vi "Periodic Tasks.vi"(8 "error in":errorcluster) -> ()   [LabVIEW 2018]
doc: "This VI runs in parallel to other tasks. It can contain as many user-defined periodic loops as you need. These can carry out PID or other sorts of timed response."
uses:
  <vilib>/Rock Robotics/WPI/Utilities/WPI_GetSetVariantRefNum.vi
  Functions/Global Variables/reset gyro.vi
  <vilib>/Rock Robotics/WPI/ThirdParty/Sensors/ADIS16448 IMU/ADIS16448_IMU.lvlib
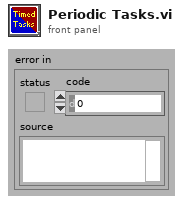
[diagram p1: front panel]
types:
  T1 = typedef "ADIS16448_IMU.lvlib/ADI_IMU_ADIS16448_IMUDevRef.ctl" = cluster{"DevStatus":errorcluster, "Handle":i32, "SPI Bus":T2, "Device Found":bool, "Device Ready":bool, "Yaw Axis":enum16{"X", "Y", "Z"}, "AHRS Algorithm":enum16{"Complementary", "Madgwick"}, "Serial":u16, "Lot ID 2":u16, "Lot ID 1":u16, "Bytes Per Sample":u16, "Calibrate On Open?":bool}
  T2 = typedef "spi_bus.ctl" = enum16{"SPI On-Board, CS0", "SPI On-Board, CS1", "SPI On-Board, CS2", "SPI On-Board, CS3", "SPI MXP", "Invalid"}
  T3 = typedef "WPI_JoystickDevRef.ctl" = cluster{"Device":T4}
  T4 = typedef "WPI_JoystickDeviceEnum.ctl" = enum16{"USB 0", "USB 1", "USB 2", "USB 3", "USB 4", "USB 5"}
  T5 = cluster{"JoystickDevRef":T3, "ADI IMU DevRef":T1}
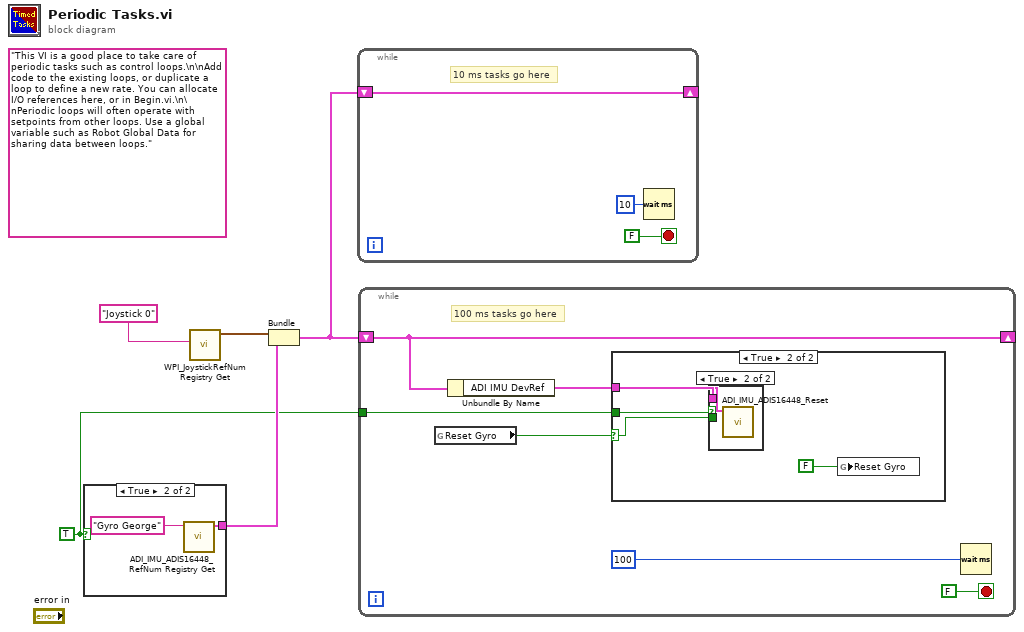
[diagram p0: block diagram]
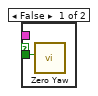
[diagram p4: hidden frame]
diagram:
  w1 = TRUE
  (unwired) "This VI is a good place to take care of periodic tasks such as control loops.\n\nAdd code to the existing loops, or duplicate a loop to define a new rate. You can allocate I/O references here, or in Begin.vi.\n\nPeriodic loops will often operate with setpoints from other loops. Use a global variable such as Robot Global Data for sharing data between loops."
  n1 = case shown="True" w1 {
    tunnel: [_ w6] -> w2
    frame False {
    }
    frame True {
      n2 = call <vilib>:"ADI_IMU_ADIS16448_RefNum Registry Get.vi"("refnum name"="Gyro George") -> ("ADI IMU DevRef"=w6:T1)  [unwired: 9 in, 1 out]
    }
  }
  n3 = call <vilib>:"WPI_JoystickRefNum Registry Get.vi"("refnum name"="Joystick 0") -> ("JoystickDevRef"=w4:T3)  [unwired: 1 in, 9 out]
  n4 = Bundle("JoystickDevRef"=w4, "ADI IMU DevRef"=w2) -> (w3:T5)  [unwired: 1 out]
  n5 = while {
    shift-right: [w8] -> _
    shift-left: w3 -> [w8]
    stop <- FALSE stop-if-true
    # "10 ms tasks go here"
    n6 = Wait (ms)(milliseconds to wait=u32 10) -> ()  [unwired: 1 out]
  }
  n7 = while {
    shift-right: [w14] -> _
    shift-left: w3 -> [w14]
    tunnel: w1 -> [w11]
    stop <- FALSE stop-if-true
    # "100 ms tasks go here"
    n8 = global read "reset gyro.vi" "Reset Gyro"() -> (w13:bool)
    n9 = Unbundle By Name(w14) -> ("ADI IMU DevRef"=w12:T1)
    n10 = case shown="True" w13 {
      selector: w13 -> [_ w18]
      tunnel: w12 -> [_ w20]
      tunnel: w11 -> [_ w17]
      frame False {
      }
      frame True {
        n11 = case shown="True" w17 {
          tunnel: w20 -> [_ w22]
          tunnel: w18 -> [w21 _]
          frame False {
            n12 = call "Zero Yaw.vi"("Zero"=w21) -> ()  [unwired: 11 in]
          }
          frame True {
            n13 = call <vilib>:"ADI_IMU_ADIS16448_Reset.vi"("ADI IMU DevRef"=w22) -> ()  [unwired: 9 in, 2 out]
          }
        }
        n14 = global write "reset gyro.vi" "Reset Gyro"(FALSE ("Reset Gyro")) -> ()
      }
    }
    n15 = Wait (ms)(milliseconds to wait=u32 100) -> ()  [unwired: 1 out]
  }
